vi "ROI group-Extract selected groups data-Core.vi"(8 "error in":errorcluster) -> (0 "Error out":errorcluster, 1 "X-axis max/min":cluster{"X-axis max":dbl, "X-axis min":dbl}, 2 "Data for ticked Groups":T1, 3 "Number of selected groups":i32)   [LabVIEW 2017]
uses:
  xcontrol/Interface VIs/Interface typedefs/Interface-Data array.ctl
  xcontrol/Interface VIs/Interface typedefs/Interface-Data format definition.ctl
  xcontrol/Typedefs/Xctl-XY data type definition.ctl
  xcontrol/Typedefs/Xctrl-ROI type enum.ctl
  Typedefs/Get-Set-Clear Control.ctl
  Global variables/gl_Functional Imaging-Global variables.vi
  xcontrol/XGrapher.xctl
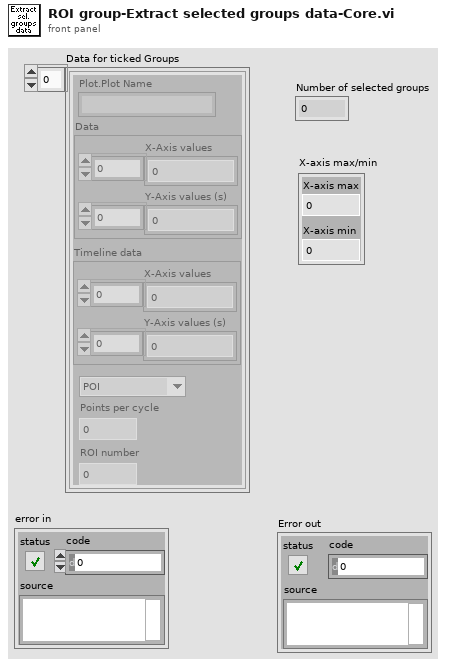
[diagram p1: front panel]
types:
  T1 = typedef "Interface-Data array.ctl" = T2[]
  T2 = typedef "Interface-Data format definition.ctl" = cluster{"Plot.Plot Name":string, "Data":T3, "Timeline data":T3, "Type":T4, "Points per cycle":u16, "ROI number":u16}
  T3 = typedef "XGrapher.xctl/Xctl-XY data type definition.ctl" = cluster{"X-Axis values":sgl[], "Y-Axis values (s)":sgl[]}
  T4 = typedef "Xctrl-ROI type enum.ctl" = enum16{"POI", "Mini-scan", "Group"}
  T5 = typedef "Get-Set-Clear Control.ctl" = enum16{"Get", "Set", "Clear"}
  T6 = typedef "Functional Imging UI Refs.ctl" = cluster{"Menu ref":refnum<k9>, "Image control":refnum<vi>, "VI ref":refnum<vi>, "XGrapher":refnum<vi>, "Smoothing":refnum<vi>, "POI Averaging":refnum<vi>, "Normalize":refnum<vi>, "POI data points in each trial":refnum<vi>, "Channel":refnum<vi>, "Experiment data folder path":refnum<vi>, "[ROI vis]":refnum<vi>, "[Groups] visbl":T7, "Group Name":refnum<vi>, "POI index":refnum<vi>, "Trial No.":refnum<vi>, "Intensity Zoom":refnum<vi>, "Trial Cursor Enabled":refnum<vi>, "Number of Trials (ind 1)":refnum<vi>, "Number of Trials (ind 2)":refnum<vi>, "MiniScans Available":refnum<vi>, "POI Available":refnum<vi>, "Defer graph updates":refnum<vi>, "Waveform selector":refnum<vi>, "#of selected POI":refnum<vi>, "#of selected MiniScans":refnum<vi>, "#of selected groups":refnum<vi>, "Max Z-Projection":refnum<vi>, "Z-Plane Selector":refnum<vi>, "Index of miniscan point to visualise":refnum<vi>, "ROI vis. mode":refnum<vi>, "Total # of points":refnum<vi>, "Index of group clicked on":refnum<vi>, "Pane 1":refnum<vi>, "Pane 2":refnum<vi>, "Pane 3":refnum<vi>, "Pane 4":refnum<vi>, "Pane 5":refnum<vi>, "Pane 6":refnum<vi>, "Deselect all ROI":refnum<vi>, "Deselect all groups":refnum<vi>}
  T7 = typedef "Groups array referecne.ctl" = refnum<vi>
  T8 = typedef "Group sel cluster.ctl" = cluster{"Group number":string, "Group Name":string, "Visibility":bool, "Highlight":bool}
  T9 = typedef "ROI group info cluster.ctl" = cluster{"Group name":string, "# ROI in group":i32, "ROI numbers in group":i32[], "Group region specifier cluster":T10}
  T10 = typedef "ROI Descriptor" = cluster{"Global Rectangle":i32[], "Contours":cluster{"ID":enum32{"External", "Internal"}, "Type":u32, "Coordinates":i32[]}[]}
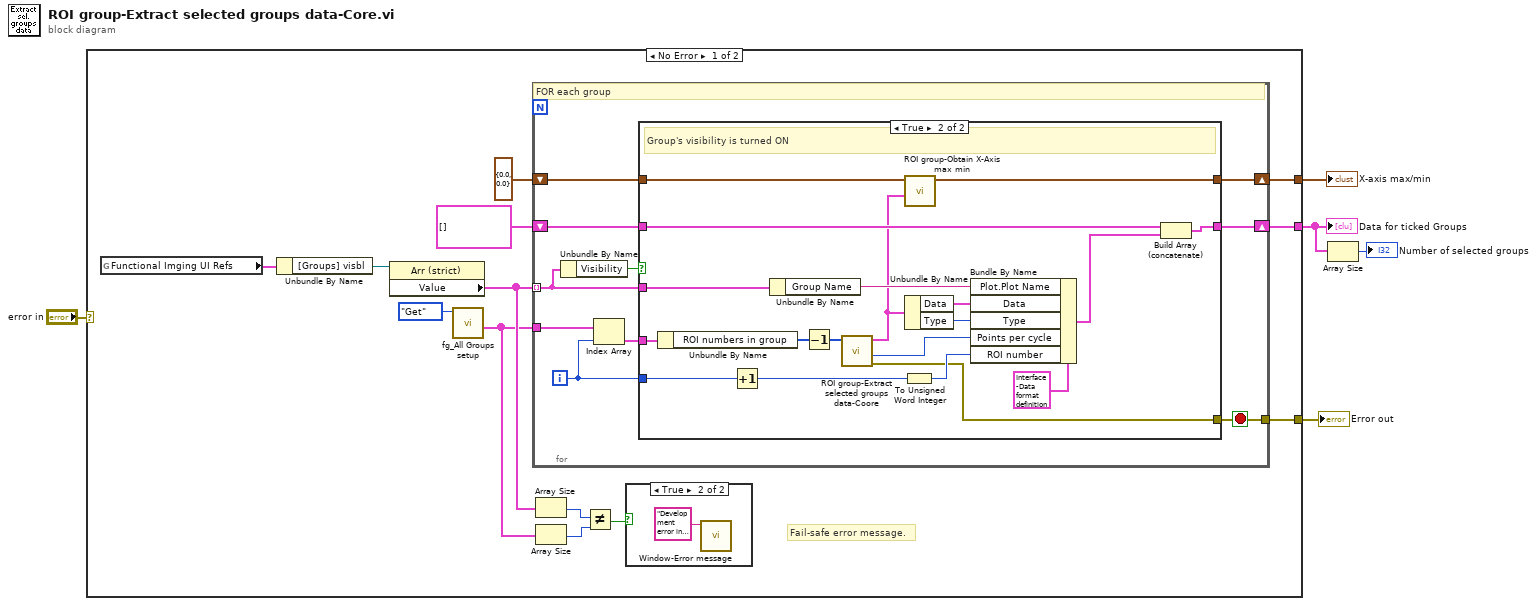
[diagram p0: block diagram]
diagram:
  n1 = case shown="No Error" "error in" {
    selector: "error in" -> [_ w51]
    tunnel: [w16 _] -> w2
    tunnel: [w7 _] -> w5
    tunnel: [w6 w51] -> w4
    frame No Error {
      # "Fail-safe error message."
      n2 = global read "gl_Functional Imaging-Global variables.vi" "Functional Imging UI Refs"() -> (w14:T6)
      n3 = Unbundle By Name(w14) -> ("[Groups] visbl"=w17:T7)
      n4 = property on="Property Node" class="Arr (strict)"(reference=w17) -> ("Value"=w13:T8[])  [unwired: 1 in, 2 out]
      n5 = call "fg_All Groups setup.vi"("Function"=Get-Set-Clear_Control."Get") -> ("Groups setup out"=w12:T9[])  [unwired: 9 in, 1 out]
      n6 = for {
        tunnel: w13 -> [w26] mode=indexing
        tunnel: w12 -> [w25]
        shift-right: [w27] -> w16
        shift-left: T1 [] ("Data for ticked Groups") -> [w28]
        shift-right: [w22] -> w7
        shift-left: cluster{"Max":dbl, "Min":dbl} {"Max"=0.0, "Min"=0.0} -> [w21]
        tunnel: [w20] -> w6
        i -> [w23]
        stop <- w20 stop-if-true
        # "FOR each group"
        n7 = Unbundle By Name(w26) -> ("Visibility"=w29:bool)
        n8 = Index Array(array=w25, index=w23) -> (element=w24:T9)
        n9 = case shown="True" w29 {
          tunnel: w24 -> [_ w50]
          tunnel: [w31 w45] -> w27
          tunnel: w28 -> [w31 w46]
          tunnel: w26 -> [_ w44]
          tunnel: w23 -> [_ w42]
          tunnel: [w30 w35] -> w22
          tunnel: w21 -> [w30 w34]
          tunnel: [_ w32] -> w20
          frame False {
            # "Group's visibility is OFF"
          }
          frame True {
            # "Group's visibility is turned ON"
            n10 = Unbundle By Name(w50) -> ("ROI numbers in group"=w43:i32[])
            n11 = Increment(x=w42) -> (x+1=w41:i32)
            n12 = Unbundle By Name(w44) -> ("Group Name"=w49:string)
            n13 = Decrement(x=w43) -> (x-1=w38:i32[])
            n14 = call "ROI group-Extract selected groups data-Coore.vi"("Indexes of ROI in group"=w38) -> ("error IO"=w32:errorcluster, "Points per cycle"=w39:u16, "ROI group data"=w33:T2)  [unwired: 8 in]
            n15 = To Unsigned Word Integer(number=w41) -> (unsigned 16bit integer=w40:u16)
            n16 = call "ROI group-Obtain X-Axis max min.vi"("ROI group data"=w33, "Max min-shift in"=w34) -> ("Max min out"=w35:cluster{dbl, dbl})  [unwired: 9 in]
            n17 = Unbundle By Name(w33) -> ("Data"=w37:T3, "Type"=w36:T4)
            n18 = Bundle By Name(cluster=T2 {"Plot.Plot Name"="", "Data"={"X-Axis values"=[], "Y-Axis values (s)"=[]}, "Timeline data"={"X-Axis values"=[], "Y-Axis values (s)"=[]}, "Type"=enum."POI", "Points per cycle"=0, "ROI number"=0}, "Plot.Plot Name"=w49, "Data"=w37, "Type"=w36, "Points per cycle"=w39, "ROI number"=w40) -> (w47:T2)
            n19 = Build Array (concatenate)(w46, w47) -> (w45:T1)
          }
        }
      }
      n20 = Array Size(array=w13) -> (size(s)=w11:i32)
      n21 = Array Size(array=w12) -> (size(s)=w10:i32)
      n22 = Not Equal?(x=w11, y=w10) -> (x != y?=w9:bool)
      n23 = case shown="True" w9 {
        frame False {
        }
        frame True {
          n24 = call "Window-Error message.vi"("Message"="Development error in the \"ROI group-Extract selected groups data-Core.vi\"\nArray mismatch.") -> ()  [unwired: 10 in, 1 out]
        }
      }
    }
    frame Error {
    }
  }
  "Data for ticked Groups" <- w2
  "X-axis max/min" <- w5
  "Error out" <- w4
  n25 = Array Size(array=w2) -> (size(s)=→"Number of selected groups":i32)
